vi "MoveSlides.vi"(2 "Min Zoom":dbl, 3 "current":T1, 4 "desired":T1={"Slide path"="", "Transition"=enum."Pan", "frame"={"left"=0, "top"=0, "right"=0, "bottom"=0}, "Number"=-1}, 5 "Map":refnum<vi>) -> (0 "index":i32, 1 "desired out":T1)   [LabVIEW 2012]
uses:
  SlideTypeDef.ctl
  LVPresent_Globals.vi
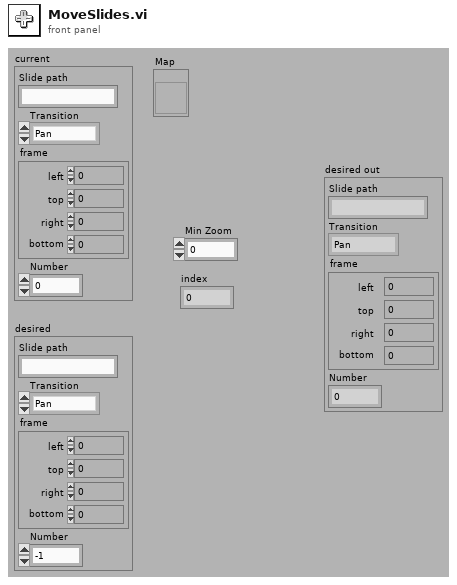
[diagram p1: front panel]
types:
  T1 = typedef "SlideTypeDef.ctl" = cluster{"Slide path":string, "Transition":enum16{"Pan", "Zoom-pan-zoom", "Zoom-wait-Zoom"}, "frame":cluster{"left":i16, "top":i16, "right":i16, "bottom":i16}, "Number":i32}
  T2 = typedef "LVPositionTypeDef.ctl" = cluster{"Left":i32, "Top":i32}
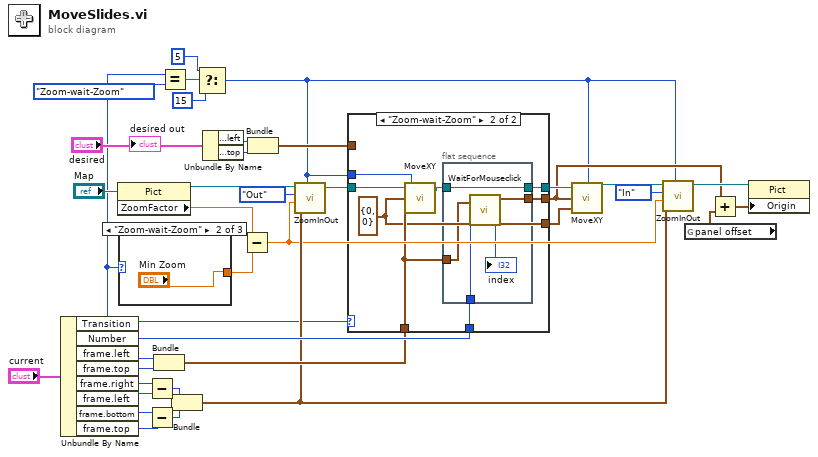
[diagram p0: block diagram]
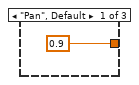
[diagram p3: hidden frame]
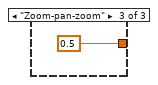
[diagram p4: hidden frame]
diagram:
  n1 = Unbundle By Name("current") -> ("Transition"=w6:enum16{"Pan", "Zoom-pan-zoom", "Zoom-wait-Zoom"}, "Number"=w26:i32, "frame.left"=w28:i16, "frame.top"=w27:i16, "frame.right"=w35:i16, "frame.left"=w34:i16, "frame.bottom"=w31:i16, "frame.top"=w32:i16)
  n2 = property class="Pict"(reference="Map") -> (reference out=w21:refnum<vi>, "ZoomFactor"=w36:sgl)  [unwired: 1 in, 1 out]
  n3 = case shown="\"Zoom-wait-Zoom\"" w6 {
    tunnel: [0.9 "Min Zoom" 0.5] -> w33
    frame "Pan", Default {
    }
    frame "Zoom-wait-Zoom" {
    }
    frame "Zoom-pan-zoom" {
    }
  }
  n4 = Subtract(x=w35, y=w34) -> (x-y=w30:i16)
  n5 = Subtract(x=w31, y=w32) -> (x-y=w29:i16)
  n6 = Bundle("left"=w28, "top"=w27) -> (w22:cluster{"left":i16, "top":i16})  [unwired: 1 in]
  n7 = Equal?(x=w6, y=enum16{"Pan", "Zoom-pan-zoom", "Zoom-wait-Zoom"}."Zoom-wait-Zoom") -> (x = y?=w4:bool)
  n8 = Bundle(w30, w29) -> (w18:cluster{i16, i16})  [unwired: 1 in]
  n9 = Select(t=5, s=w4, f=15) -> (s? t:f=w1:i32)
  n10 = Unbundle By Name("desired") -> ("frame.left"=w14:i16, "frame.top"=w13:i16)
  n11 = Subtract(x=w36, y=w33) -> (x-y=w16:dbl)
  n12 = Bundle("left"=w14, "top"=w13) -> (w11:cluster{"left":i16, "top":i16})  [unwired: 1 in]
  n13 = call "ZoomInOut.vi"("Map in"=w21, "Direction"=enum16{"Out", "In"}."Out", "Zoom diff"=w16, "Image Size"=w18, "Iterations"=w1) -> ("Map out"=w20:refnum<vi>)  [unwired: 2 in]
  n14 = case shown="\"Zoom-wait-Zoom\"" w6 {
    tunnel: [w43 w45] -> w24
    tunnel: w20 -> [w43 w48]
    tunnel: w22 -> [w42 w47]
    tunnel: [w41 w51] -> w7
    tunnel: w26 -> [_ w50]
    tunnel: w1 -> [_ w49]
    tunnel: [w42 w46] -> w23
    tunnel: w11 -> [w41 _]
    frame Default {
    }
    frame "Zoom-wait-Zoom" {
      w46 = cluster{"left":i16, "top":i16} {"left"=0, "top"=0} ("Desired")
      n15 = call "MoveXY.vi"("Iterations"=w49, "Current"=w47, "Desired"=w46, "Map in"=w48) -> ("Map out"=w44:refnum<vi>)  [unwired: 1 out]
      n16 = flat-sequence {
        tunnel: [w56] -> w51
        tunnel: w50 -> [w55]
        tunnel: w47 -> [w53]
        tunnel: [w52] -> w45
        tunnel: w44 -> [w52]
        frame #0 {
          n17 = call "WaitForMouseclick.vi"("index In"=w55, "Origin"=w53) -> ("index"=→"index":i32, "Dest"=w56:cluster{"left":i16, "top":i16})
        }
      }
    }
  }
  n18 = call "MoveXY.vi"("Iterations"=w1, "Current"=w23, "Desired"=w7, "Map in"=w24) -> ("Map out"=w19:refnum<vi>)  [unwired: 1 out]
  n19 = call "ZoomInOut.vi"("Map in"=w19, "Direction"=enum16{"Out", "In"}."In", "Zoom diff"=w16, "Image Size"=w18, "Iterations"=w1) -> ("Map out"=w8:refnum<vi>)  [unwired: 2 in]
  n20 = global read "LVPresent_Globals.vi" "panel offset"() -> (w10:T2)
  n21 = Add(x=w7, y=w10) -> (x+y=w9:T2)
  n22 = property class="Pict"(reference=w8, "Origin"=w9) -> ()  [unwired: 1 in, 2 out]
  "desired out" <- "desired"
